vi "Helper SubVI - Signal Sweep (tsa).vi"(8 "reset":bool, 9 "length":i32=-1, 10 "shift (%)":dbl=25.0, 11 "Signal in":waveform(dbl)={"t0"=timestamp(0 s since 1904-01-01), "dt"=0.0, "Y"=[]}) -> (3 "Signal out":waveform(dbl))   [LabVIEW 2023]
doc: "Rotates the signal or gets a subset from the input signal."
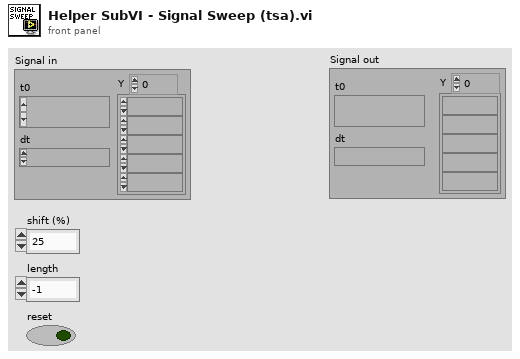
[diagram p1: front panel]
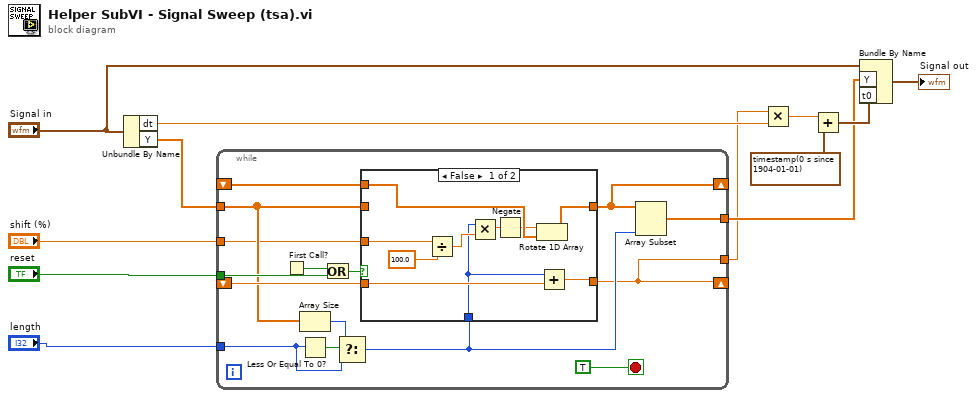
[diagram p0: block diagram]
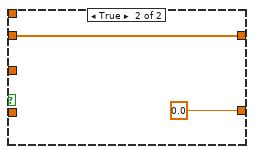
[diagram p2: hidden frame]
diagram:
  n1 = Unbundle By Name("Signal in") -> ("dt"=w10:dbl, "Y"=w1:dbl[])
  n2 = while {
    shift-right: [w20] -> _
    shift-left: _ -> [w24]
    shift-right: [w13] -> _
    shift-left: _ -> [w19]
    tunnel: "reset" -> [w18]
    tunnel: w1 -> [w17]
    tunnel: "shift (%)" -> [w16]
    tunnel: "length" -> [w15]
    tunnel: [w14] -> w3
    tunnel: [w13] -> w2
    stop <- TRUE stop-if-true
    n3 = First Call?() -> (First Call?: T/F=w27:bool)
    n4 = Array Size(array=w17) -> (size(s)=w22:i32)
    n5 = Less Or Equal To 0?(x=w15) -> (x <= 0?=w23:bool)
    n6 = Or(x=w27, y=w18) -> (x .or. y?=w26:bool)
    n7 = Select(t=w22, s=w23, f=w15) -> (s? t:f=w21:i32)
    n8 = case shown="False" w26 {
      tunnel: w17 -> [_ w39]
      tunnel: [w37 w39] -> w20
      tunnel: w24 -> [w34 _]
      tunnel: w21 -> [w29 _]
      tunnel: [w32 0.0] -> w13
      tunnel: w19 -> [w31 _]
      tunnel: w16 -> [w28 _]
      frame False {
        n9 = Divide(x=w28, y=100.0) -> (x/y=w36:dbl)
        n10 = Multiply(x=w29, y=w36) -> (x*y=w33:dbl)
        n11 = Negate(x=w33) -> (-x=w30:dbl)
        n12 = Rotate 1D Array(1:w34, 2:w30) -> (0:w37:dbl[])
        n13 = Add(x=w29, y=w31) -> (x+y=w32:dbl)
      }
      frame True {
      }
    }
    n14 = Array Subset(array=w20, length=w21) -> (w14:dbl[])  [unwired: 1 in]
  }
  n15 = Multiply(x=w2, y=w10) -> (x*y=w9:dbl)
  n16 = Add(x=w9, y=timestamp(0 s since 1904-01-01) ("t0")) -> (x+y=w7:timestamp)
  n17 = Bundle By Name(cluster="Signal in", "Y"=w3, "t0"=w7) -> (→"Signal out":waveform(dbl))
